vi "Initialize.vi"(8 "error in (no error)":errorcluster, 11 "Simulated Detector in":refnum<class "Simulated Detector.lvclass">) -> (0 "error out":errorcluster, 3 "Simulated Detector out":refnum<class "Simulated Detector.lvclass">)   [LabVIEW 2019, in "Simulated Detector.lvclass"]
uses:
  Simulated Detector.lvclass
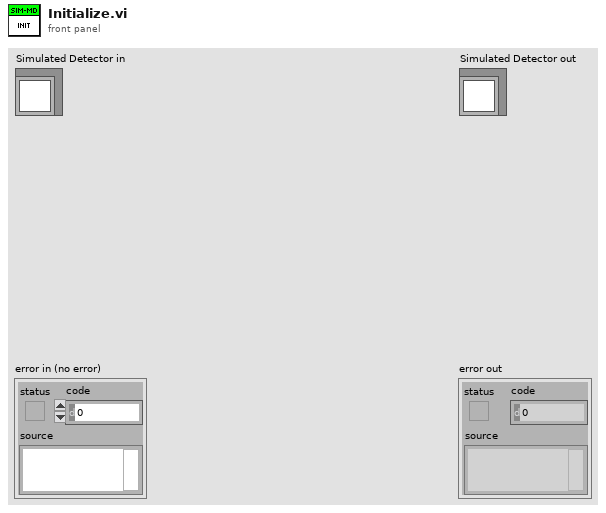
[diagram p1: front panel]
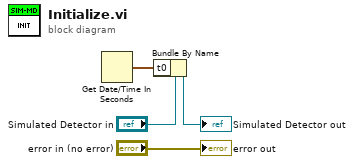
[diagram p0: block diagram]
diagram:
  n1 = Get Date/Time In Seconds() -> (seconds since 1Jan1904=w1:timestamp)
  n2 = Bundle By Name(cluster="Simulated Detector in", "t0"=w1) -> (→"Simulated Detector out":refnum<class "Simulated Detector.lvclass">)
  "error out" <- "error in (no error)"
